vi "Read Protected Subpanel.vi"(8 "error in (no error)":errorcluster, 11 "View Manager in":refnum<class "View Manager.lvclass">=refnum) -> (0 "error out":errorcluster, 2 "Protected Subpanel":T1, 3 "View Manager out":refnum<class "View Manager.lvclass">)   [LabVIEW 2017, in "View Manager.lvlib" / "View Manager.lvclass"]
uses:
  View Manager.lvclass
  <vilib>/gpm_packages/@cs/mva-viewable/Source/IViewable/ProtectedSubpanel/ProtectedSubpanel.lvclass
  <vilib>/gpm_packages/@cs/mva-viewable/Source/IViewable/ProtectedSubpanel/Protected Subpanel Reference.ctl
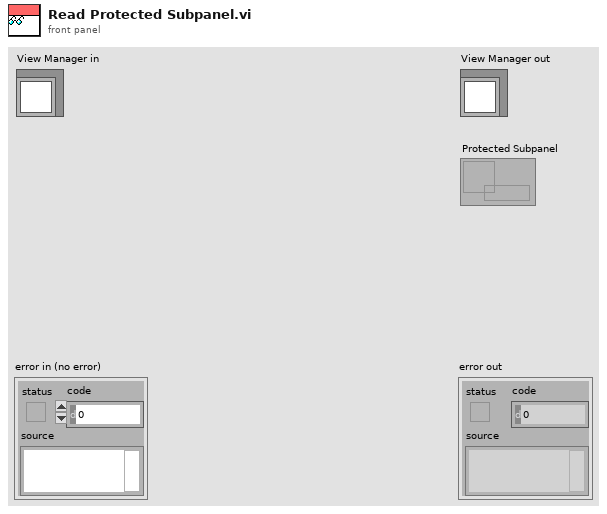
[diagram p1: front panel]
types:
  T1 = typedef "IViewable.lvlib/ProtectedSubpanel.lvclass/Protected Subpanel Reference.ctl" = refnum<data-value>
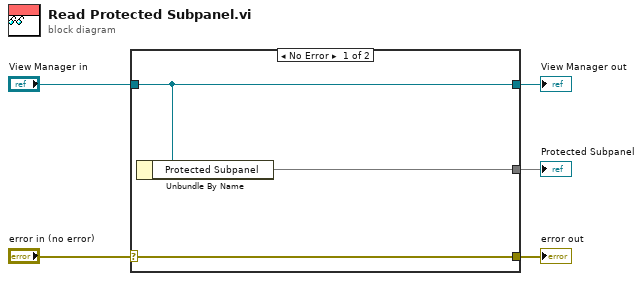
[diagram p0: block diagram]
diagram:
  n1 = case shown="No Error" "error in (no error)" {
    selector: "error in (no error)" -> [w8 w9]
    tunnel: [w8 w9] -> w4
    tunnel: [w7 w10] -> w2
    tunnel: "View Manager in" -> [w7 w10]
    tunnel: [w6 _] -> w1
    frame No Error {
      n2 = Unbundle By Name(w7) -> ("Protected Subpanel"=w6)
    }
    frame Error {
    }
  }
  "error out" <- w4
  "View Manager out" <- w2
  "Protected Subpanel" <- w1
